vi "sub build title.vi"(8 "error in":errorcluster, 11 "frame title":T1={"number"="", "name"="-"}) -> (0 "error out":errorcluster, 3 "title string":string)   [LabVIEW 2018, in "Data Parser.lvclass"]
uses:
  Data Parser.lvclass
  frame title.ctl
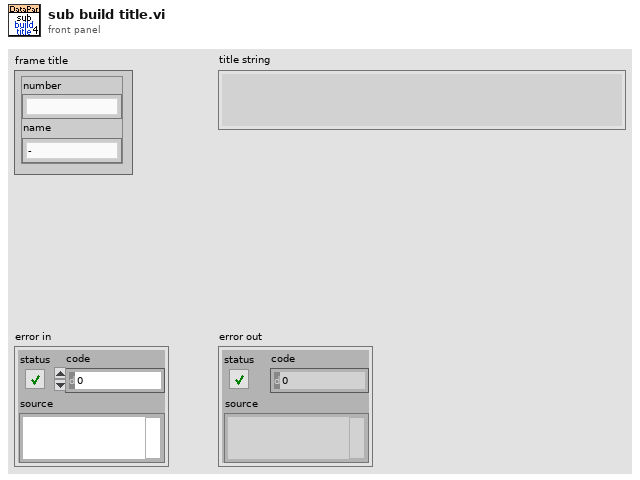
[diagram p1: front panel]
types:
  T1 = typedef "Data Parser.lvclass/frame title.ctl" = cluster{"number":string, "name":string}
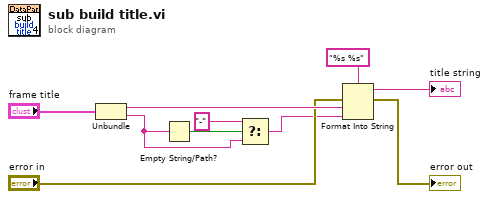
[diagram p0: block diagram]
diagram:
  n1 = Unbundle("frame title") -> ("number"=w8:string, "name"=w3:string)
  n2 = Empty String/Path?(string/path=w3) -> (empty?=w4:bool)
  n3 = Select(t="-", s=w4, f=w3) -> (s? t:f=w2:string)
  n4 = Format Into String(format string="%s %s", error in="error in", w8, w2) -> (resulting string=→"title string":string, error out=→"error out":errorcluster)  [unwired: 1 in]
